vi "square-of-sum.vi"(8 "error in (no error)":errorcluster, 11 "Input integers":i64[](array[numeric])=[1, 2, 3, 4, 5, 6, 7, 8, 9, 10]) -> (0 "error out":errorcluster, 3 "square-of-sum":i64)   [LabVIEW 2021, in "Project Euler.lvlib"]
uses:
  Project Euler.lvlib
panel:
  # "Development\ncontrols/indicators useful for development and testing, but which are not outputs of the VI"
  # "Input\nInputs to the VI"
  # "Output\nOutputs of the VI"
  # "Description\n\nBlank VI with error handling case. \n\nSummarize the use of this VI in this space."
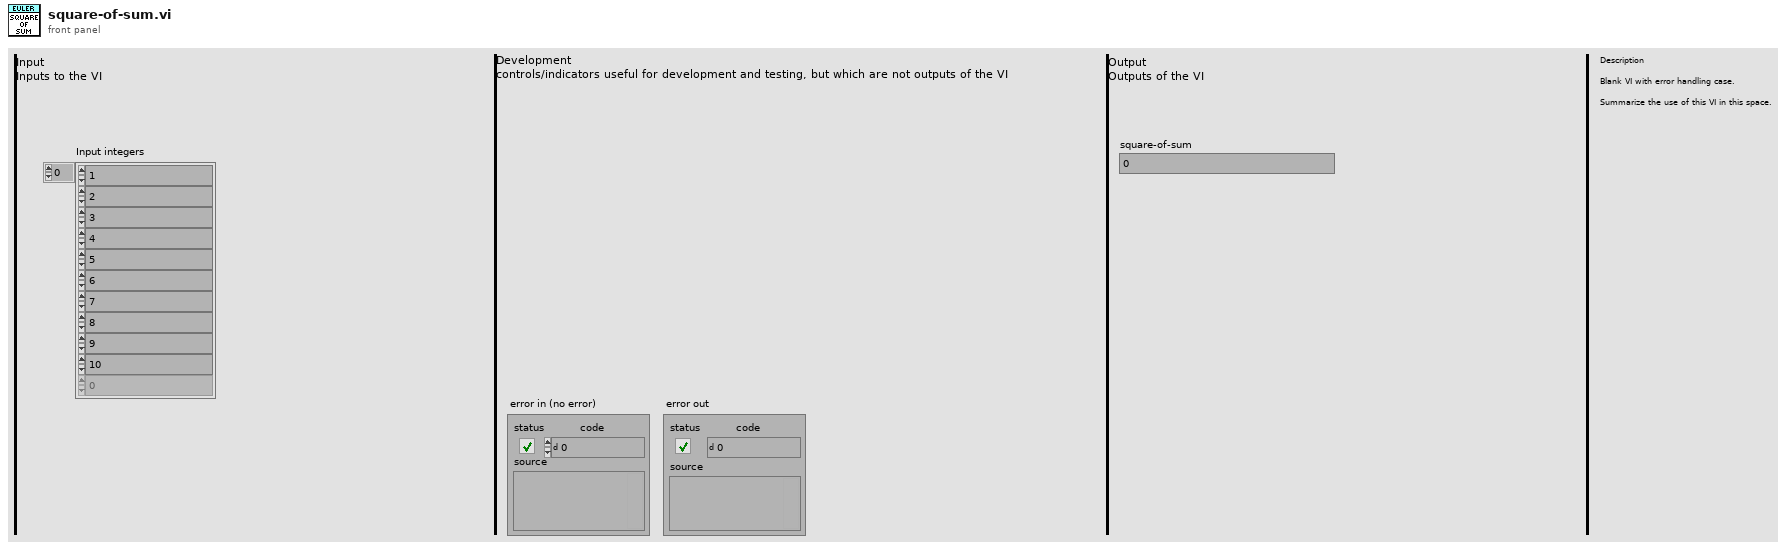
[diagram p1: front panel]
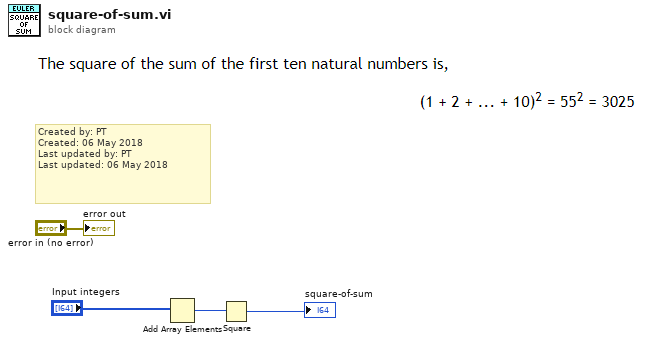
[diagram p0: block diagram]
diagram:
  # "Created by: PT\nCreated: 06 May 2018\nLast updated by: PT\nLast updated: 06 May 2018"
  n1 = Add Array Elements(numeric array="Input integers") -> (sum=w2:i64)
  n2 = Square(x=w2) -> (x^2=→"square-of-sum":i64)
  "error out" <- "error in (no error)"
